vi "(5) Encoder Version Movement.vi"(3 "Move":bool) -> ()   [LabVIEW 2020]
uses:
  <instrlib>/Arcus Ethernet Driver 1.0.0/ArcusEthernetComm/classes/Controller/_Controller.lvclass
panel:
  out "Scanning Rig Disconnection":errorcluster={"status"=TRUE, "code"=0, "source"=""}
  in  "error in (no error)":errorcluster
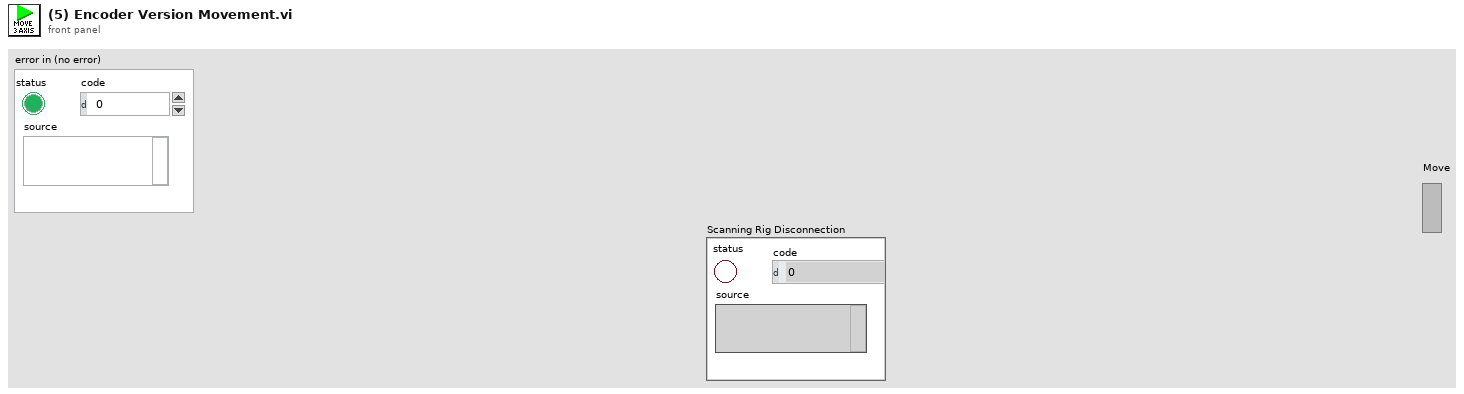
[diagram p1: front panel]
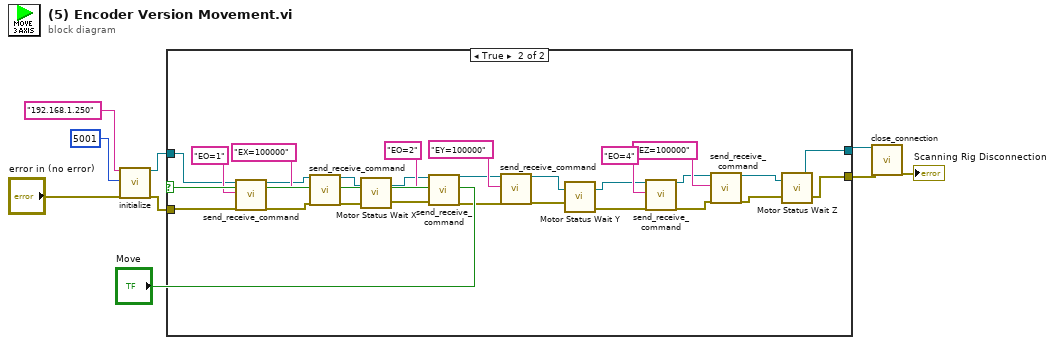
[diagram p0: block diagram]
diagram:
  n1 = call <instrlib>:"initialize.vi"("ip_address (in)"="192.168.1.250", "dev_port(def=5001)"=u16 5001, "error in (no error)"="error in (no error)") -> ("reference (out)"=w5:refnum<class "_Controller.lvclass">, "error out"=w4:errorcluster)  [unwired: 15 in]
  n2 = case shown="True" "Move" {
    tunnel: w5 -> [w11 w13]
    tunnel: w4 -> [w10 w14]
    tunnel: [w11 w28] -> w2
    tunnel: [w10 w29] -> w1
    frame False {
    }
    frame True {
      n3 = call <instrlib>:"send_receive_command.vi"("reference (in)"=w13, "ASCII Command (in)"="EO=1", "error in (no error)"=w14) -> ("reference (out)"=w15:refnum<class "_Controller.lvclass">, "error out"=w12:errorcluster)  [unwired: 12 in, 3 out]
      n4 = call <instrlib>:"send_receive_command.vi"("reference (in)"=w15, "ASCII Command (in)"="EX=100000", "error in (no error)"=w12) -> ("reference (out)"=w17:refnum<class "_Controller.lvclass">, "error out"=w16:errorcluster)  [unwired: 12 in, 3 out]
      n5 = call "Motor Status Wait X.vi"("error in"=w16, "reference (in)"=w17) -> ("error out"=w19:errorcluster, "reference (out)"=w18:refnum<class "_Controller.lvclass">)
      n6 = call <instrlib>:"send_receive_command.vi"("reference (in)"=w18, "ASCII Command (in)"="EO=2", "error in (no error)"=w19) -> ("reference (out)"=w21:refnum<class "_Controller.lvclass">, "error out"=w20:errorcluster)  [unwired: 12 in, 3 out]
      n7 = call <instrlib>:"send_receive_command.vi"("reference (in)"=w21, "ASCII Command (in)"="EY=100000", "error in (no error)"=w20) -> ("reference (out)"=w23:refnum<class "_Controller.lvclass">, "error out"=w22:errorcluster)  [unwired: 12 in, 3 out]
      n8 = call "Motor Status Wait Y.vi"("error in"=w22, "reference (in)"=w23) -> ("error out 2"=w27:errorcluster, "reference (out) 2"=w26:refnum<class "_Controller.lvclass">)
      n9 = call <instrlib>:"send_receive_command.vi"("reference (in)"=w26, "ASCII Command (in)"="EO=4", "error in (no error)"=w27) -> ("reference (out)"=w25:refnum<class "_Controller.lvclass">, "error out"=w24:errorcluster)  [unwired: 12 in, 3 out]
      n10 = call <instrlib>:"send_receive_command.vi"("reference (in)"=w25, "ASCII Command (in)"="EZ=100000", "error in (no error)"=w24) -> ("reference (out)"=w31:refnum<class "_Controller.lvclass">, "error out"=w30:errorcluster)  [unwired: 12 in, 3 out]
      n11 = call "Motor Status Wait Z.vi"("error in"=w30, "reference (in)"=w31) -> ("error out 2"=w29:errorcluster, "reference (out) 2"=w28:refnum<class "_Controller.lvclass">)
    }
  }
  n12 = call <instrlib>:"close_connection.vi"("reference (in)"=w2, "error in (no error)"=w1) -> ("error out"=→"Scanning Rig Disconnection":errorcluster)  [unwired: 16 in, 1 out]
